vi "Set Timer (Quick).vi"(7 "Quick Timer":T1 {"Set-Time (s)" format="%<%H:%M>t"}, 8 "error in (no error)":errorcluster, 10 "Address (0)":i32, 11 "VISA resource name":refnum<visa-resource-name>) -> (0 "error out":errorcluster, 3 "VISA resource name out":refnum<visa-resource-name>)   [LabVIEW 2016, in "Environment Chamber.lvlib" / "Climatic Chamber.lvlib"]
doc: "<b>Timer writing</B>\n\nEdits the quick timer."
uses:
  Climatic Chamber.lvlib
  Private/Type Defs/QuickTimer Cluster.ctl
  Private/Type Defs/Operation_Stop Mode Enum.ctl
  Private/Type Defs/TimerNumber Enum.ctl
panel:
  out "Error":bool
  out "NACK":bool
  out "ACK":bool
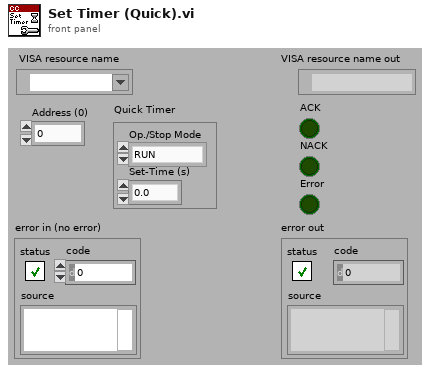
[diagram p1: front panel]
types:
  T1 = typedef "Environment Chamber.lvlib/Climatic Chamber.lvlib/QuickTimer Cluster.ctl" = cluster{"Op./Stop Mode":T2, "Set-Time (s)":dbl}
  T2 = typedef "Environment Chamber.lvlib/Climatic Chamber.lvlib/Operation_Stop Mode Enum.ctl" = enum16{"RUN", "CONSTANT", "STANDBY", "OFF"}
  T3 = typedef "Environment Chamber.lvlib/Climatic Chamber.lvlib/TimerNumber Enum.ctl" = enum16{"Quick Timer", "Start Timer", "End Timer"}
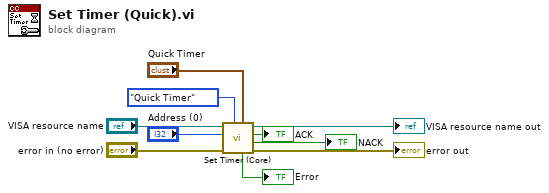
[diagram p0: block diagram]
diagram:
  n1 = call "Set Timer (Core).vi"("Quick Timer"="Quick Timer", "Timer Number"=TimerNumber_Enum."Quick Timer", "error in (no error)"="error in (no error)", "Address (0)"="Address (0)", "VISA resource name"="VISA resource name") -> ("error out"=→"error out":errorcluster, "NACK"=→"NACK":bool, "ACK"=→"ACK":bool, "VISA resource name out"=→"VISA resource name out":refnum<visa-resource-name>, "Error"=→"Error":bool)  [unwired: 2 in]
